vi "MotionProfiles_SendTraj.vi"(8 "error in (no error)":errorcluster, 11 "MotionProfiles in":refnum<class "MotionProfiles.lvclass">) -> (0 "error out":errorcluster, 3 "MotionProfiles out":refnum<class "MotionProfiles.lvclass">)   [LabVIEW 2016, in "MotionProfiles.lvclass"]
uses:
  MotionProfiles.lvclass
  MotionProfiles.lvclass/MotionProfiles.ctl
  <vilib>/Rock Robotics/WPI/ThirdParty/CanMotor/TalonSRX/WPI_CANTalonSRX_MotionProfileTrajectoryPt.ctl
  <vilib>/Rock Robotics/WPI/ThirdParty/CanMotor/TalonSRX/WPI_CANTalonSRX_Params.ctl
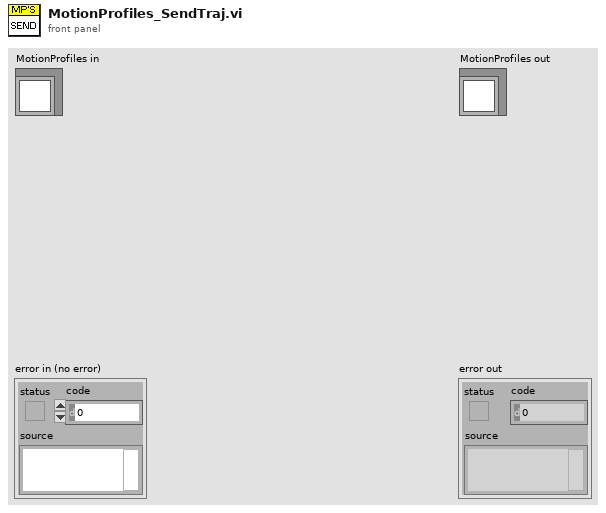
[diagram p1: front panel]
types:
  T1 = typedef "WPI_CANTalonSRX_MotionProfileTrajectoryPt.ctl" = cluster{"Duration Ms":u8, "Velocity":dbl, "Position":dbl, "Profile Slot Select":u8, "Is Last":bool, "Velocity Only":bool, "Zero Position":bool, "Compress Code":u8, "Same Velocity":i32, "Delta Position":i32, "Count":u8}
  T2 = typedef "WPI_MotorControlDeviceRef.ctl" = cluster{"DeviceStatus":errorcluster, "Type":T3, "PWM":cluster{"PWM Channel":T4, "DeadBand":T5}, "CAN":cluster{"Device Number":u8, "SetOutput VI Ref":variant, "GetOutput VI Ref":variant, "Enable VI Ref":variant, "Disable VI Ref":variant, "Data":variant}, "Invert":bool}
  T3 = typedef "WPI_MotorControlType.ctl" = enum16{"PWM", "CAN"}
  T4 = typedef "FPGA_DIOPWMChannel.ctl" = enum8{"PWM 0", "PWM 1", "PWM 2", "PWM 3", "PWM 4", "PWM 5", "PWM 6", "PWM 7", "PWM 8", "PWM 9", "PWM MXP 0", "PWM MXP 1", "PWM MXP 2", "PWM MXP 3", "PWM MXP 4", "PWM MXP 5", "PWM MXP 6", "PWM MXP 7", "PWM MXP 8", "PWM MXP 9", "Invalid"}
  T5 = typedef "WPI_PWMDeadband.ctl" = cluster{"Name":string, "maxPositivePwm":i32, "minPositivePwm":i32, "centerPwm":i32, "maxNegativePwm":i32, "minNegativePwm":i32, "angularRange":u16}
  T6 = typedef "WPI_CANTalonSRX_Params.ctl" = u8
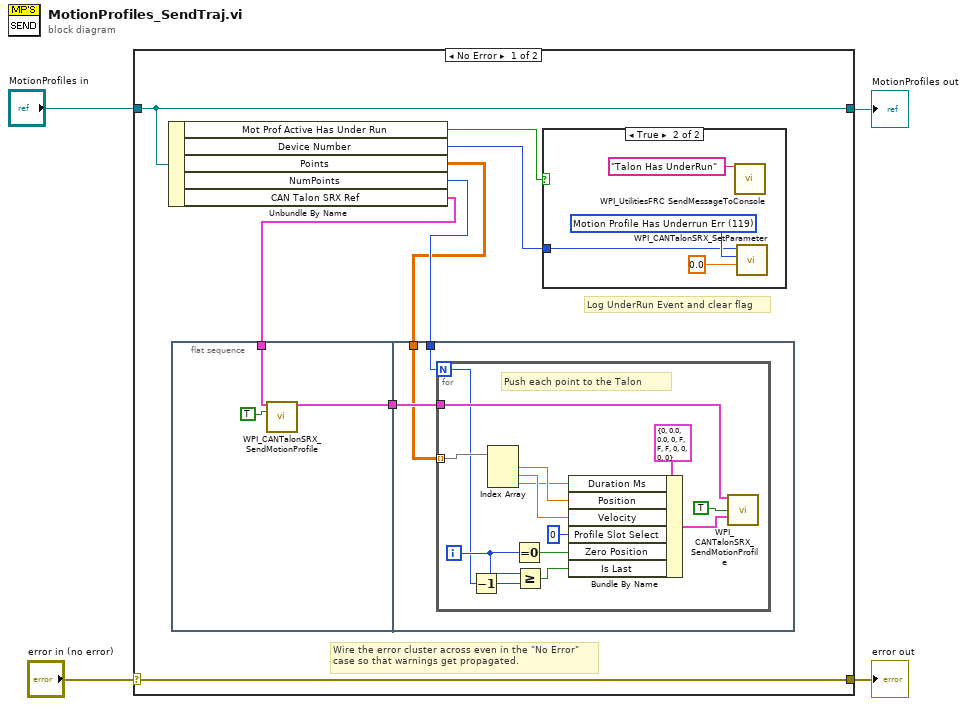
[diagram p0: block diagram]
diagram:
  n1 = case shown="No Error" "error in (no error)" {
    selector: "error in (no error)" -> [w12 w38]
    tunnel: [w12 w38] -> w3
    tunnel: [w11 w37] -> w1
    tunnel: "MotionProfiles in" -> [w11 w37]
    frame No Error {
      # "Log UnderRun Event and clear flag"
      # "Wire the error cluster across even in the \"No Error\"\ncase so that warnings get propagated."
      n2 = Unbundle By Name(w11) -> ("Mot Prof Active Has Under Run"=w10:bool, "Device Number"=w9:u8, "Points"=w5:dbl[][], "NumPoints"=w7:u16, "CAN Talon SRX Ref"=w8:T2)
      n3 = flat-sequence {
        tunnel: w8 -> [w14]
        tunnel: [w13] -> w6
        tunnel: w7 -> [w18]
        tunnel: w6 -> [w17]
        tunnel: w5 -> [w16]
        frame #0 {
          n4 = call <vilib>:"WPI_CANTalonSRX_SendMotionProfile.vi"("CAN Talon SRX Ref"=w14, "Clear"=TRUE) -> ("CAN Talon SRX Ref Out"=w13:T2)  [unwired: 10 in, 3 out]
        }
        frame #1 {
          n5 = for {
            N: w18 -> [w19]
            tunnel: w17 -> [w29]
            tunnel: w16 -> [w28] mode=indexing
            i -> [w21]
            # "Push each point to the Talon"
            n6 = Decrement(x=w19) -> (x-1=w20:i32)
            n7 = Index Array(array=w28) -> (element #1=w27:dbl, element #2=w26:dbl, element #3=w25:dbl)  [unwired: 3 in]
            n8 = Equal To 0?(x=w21) -> (x = 0?=w23:bool)
            n9 = Greater Or Equal?(x=w21, y=w20) -> (x >= y?=w22:bool)
            n10 = Bundle By Name(cluster=T1 {"Duration Ms"=0, "Velocity"=0.0, "Position"=0.0, "Profile Slot Select"=0, "Is Last"=FALSE, "Velocity Only"=FALSE, "Zero Position"=FALSE, "Compress Code"=0, "Same Velocity"=0, "Delta Position"=0, "Count"=0} ("New Point"), "Duration Ms"=w25, "Position"=w27, "Velocity"=w26, "Profile Slot Select"=u8 0, "Zero Position"=w23, "Is Last"=w22) -> (w30:T1)
            n11 = call <vilib>:"WPI_CANTalonSRX_SendMotionProfile.vi"("CAN Talon SRX Ref"=w29, "Push"=TRUE, "New Point"=w30) -> ()  [unwired: 9 in, 4 out]
          }
        }
      }
      n12 = case shown="True" w10 {
        tunnel: w9 -> [_ w33]
        frame False {
        }
        frame True {
          w35 = T6 119 items=["Slot 0 - P"=1, "Slot 0 - I"=2, "Slot 0 - D"=3, "Slot 0 - F"=4, "Slot 0 - I Zone"=5, "Slot 0 - Ramp Rate"=6, "Slot 1 - P"=11, "Slot 1 - I"=12, "Slot 1 - D"=13, "Slot 1 - F"=14, "Slot 1 - I Zone"=15, "Slot 1 - Ramp Rate"=16, "Soft Limit - Forward"=21, "Soft Limit - Reverse"=22, "Soft Limit - Forward Enable"=23, "Soft Limit - Reverse Enable"=24, "On Boot - Brake Mode"=31, "On Boot - Limit Normally Closed - Forward"=32, "On Boot - Limit Normally Closed - Reverse"=33, "On Boot - Limit Disabled - Forward"=34, "On Boot - Limit Disabled - Reverse"=35, "Fault - Over Temp"=41, "Fault - Under Voltage"=42, "Fault - Forward Limit"=43, "Fault - Reverse Limit"=44, "Fault - Hardware Failure"=45, "Fault - Forward Soft Limit"=46, "Fault - Reverse Soft Limit"=47, "Sticky Fault - Over Temp"=48, "Sticky Fault - Under Voltage"=49, "Sticky Fault - Forward Limit"=50, "Sticky Fault - Reverse Limit"=51, "Sticky Fault - Forward Soft Limit"=52, "Sticky Fault - Reverse Soft Limit"=53, "Applied Throttle"=61, "Closed-Loop Error"=62, "Select Feedback Device"=63, "Reverse Closed-Loop Output"=64, "Mode Select"=65, "Profile Slot Select"=66, "Ramp Throttle"=67, "Reverse Feedback Sensor"=68, "Limit Switch Enabled"=69, "Limit Switch Closed - Forward"=70, "Limit Switch Closed - Reverse"=71, "Sensor Position"=73, "Sensor Velocity"=74, "Current"=75, "Brake is Enabled"=76, "Encoder Position"=77, "Encoder Velocity"=78, "Encoder Index Rise Events"=79, "Encoder A Pin State"=80, "Encoder B Pin State"=81, "Encoder Index Pin State"=82, "Analog In with Overflow"=83, "Analog In Velocity"=84, "Temperature"=85, "Battery Voltage"=86, "Reset Count"=87, "Reset Flags"=88, "Firmware Version"=89, "Settings Changed"=90, "Quad Filter Enable"=91, "Ignore Disable Broadcast"=92, "I Accumulator"=93, "Status 1 Frame Rate Ms"=94, "Status 2 Frame Rate Ms"=95, "Status 3 Frame Rate Ms"=96, "Status 4 Frame Rate Ms"=97, "Status 6 Frame Rate Ms"=98, "Status 7 Frame Rate Ms"=99, "Enable Index Pin Clear Position"=100, "Peak Positive Output"=104, "Nominal Positive Output"=105, "Peak Negative Output"=106, "Nominal Negative Output"=107, "Quad Index Pin Polarity"=108, "Status 8 Frame Rate Ms"=109, "Allow Position Overflow"=110, "Slot 0 - Allowable Closed-Loop Error"=111, "Number Potentiometer Turns"=112, "Encoder Codes Per Rev"=113, "Pulse Width Decoded Position"=114, "Analog Position"=115, "Voltage Compensation Rate (V/s)"=116, "Slot 1 - Allowable Closed-Loop Error"=117, "Motion Profile Has Underrun Err"=119] ("Talon SRX Parameters")
          n13 = call <vilib>:"WPI_UtilitiesFRC SendMessageToConsole.vi"("Message"="Talon Has UnderRun") -> ()  [unwired: 14 in, 1 out]
          n14 = call <vilib>:"WPI_CANTalonSRX_SetParameter.vi"("Value"=0.0, "Parameter"=w35, "Device ID (0)"=w33) -> ()  [unwired: 7 in, 2 out]
        }
      }
    }
    frame Error {
    }
  }
  "error out" <- w3
  "MotionProfiles out" <- w1
